vi "Action Single Trigger.vi"(8 "error in (no error)":errorcluster, 11 "U2000 in":refnum<class "U2000.lvclass">) -> (0 "error out":errorcluster, 3 "U2000 out":refnum<class "U2000.lvclass">)   [LabVIEW 2020, in "U2000.lvclass"]
uses:
  U2000.lvclass
  C:/Sandbox/RF Bench/Source Code/WiSpry Test Framework/Instruments/Instrument.lvclass
  Instrument.lvclass/Instrument.ctl
  <instrlib>/Agilent U2000 Series/Agilent U2000 Series.lvlib
  Instrument.lvclass
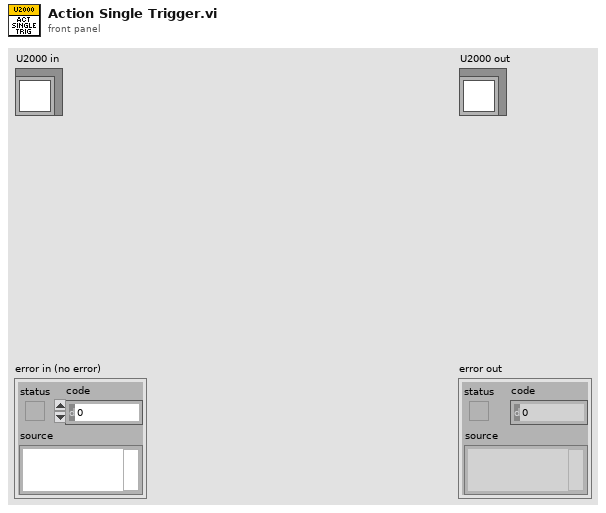
[diagram p1: front panel]
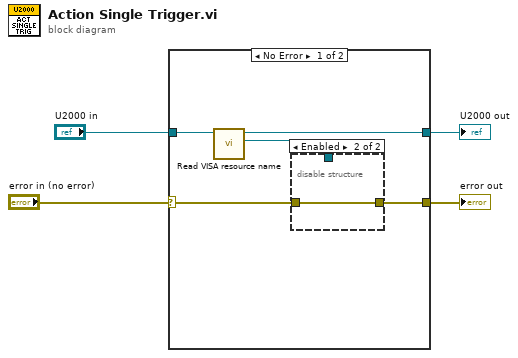
[diagram p0: block diagram]
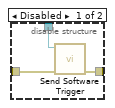
[diagram p2: hidden frame]
diagram:
  n1 = case shown="No Error" "error in (no error)" {
    selector: "error in (no error)" -> [w5 w15]
    tunnel: "U2000 in" -> [w9 w14]
    tunnel: [w8 w14] -> w3
    tunnel: [w7 w15] -> w2
    frame No Error {
      n2 = call "Read VISA resource name.vi"("Instrument in"=w9) -> ("VISA resource name"=w6:refnum<visa-resource-name>, "Instrument out"=w8:refnum<class "U2000.lvclass">)  [unwired: 9 in]
      n3 = disable-structure shown="Enabled" {
        disable-tunnel: [w12 w13] -> w7
        disable-tunnel: w6 -> [w11 _]
        disable-tunnel: w5 -> [w10 w13]
        frame Disabled {
          n4 = call <instrlib>:"Send Software Trigger.vi"("error in (no error)"=w10, "VISA resource name"=w11) -> ("error out"=w12:errorcluster)  [unwired: 8 in, 1 out]
        }
        frame Enabled {
        }
      }
    }
    frame Error {
    }
  }
  "error out" <- w2
  "U2000 out" <- w3
